vi "SimpleCalculator.vi"(1 "Operation":enum16{"ADD", "SUBTRACT", "MULTIPLY", "DIVIDE"}(ring), 2 "Number 2":dbl, 3 "Number 1":dbl) -> (0 "Result":dbl)   [LabVIEW 2020]
doc: "Simple calculator. Perform one form four mathematical operation on two numbers. Comments in polish language."
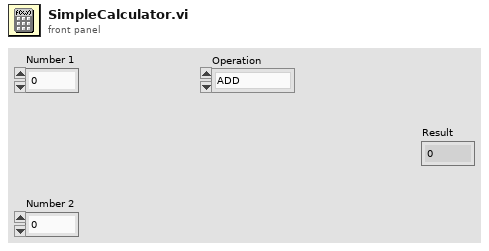
[diagram p1: front panel]
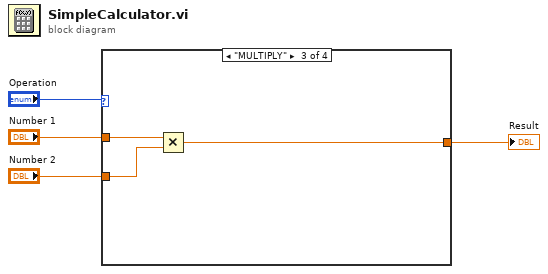
[diagram p0: block diagram]
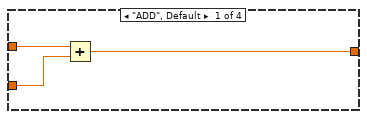
[diagram p2: hidden frame]
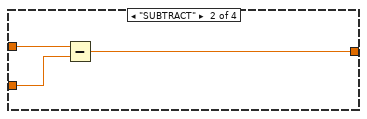
[diagram p3: hidden frame]
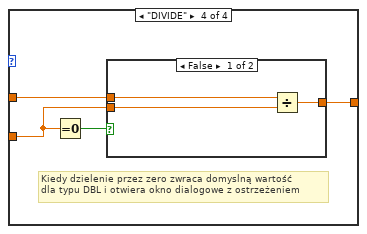
[diagram p4: hidden frame]
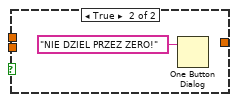
[diagram p5: hidden frame]
diagram:
  n1 = case shown="\"MULTIPLY\"" "Operation" {
    tunnel: "Number 1" -> [w7 w10 w13 w17]
    tunnel: "Number 2" -> [w6 w9 w12 w15]
    tunnel: [w5 w8 w11 w16] -> w1
    frame "ADD", Default {
      n2 = Add(x=w7, y=w6) -> (x+y=w5:dbl)
    }
    frame "SUBTRACT" {
      n3 = Subtract(x=w10, y=w9) -> (x-y=w8:dbl)
    }
    frame "MULTIPLY" {
      n4 = Multiply(x=w13, y=w12) -> (x*y=w11:dbl)
    }
    frame "DIVIDE" {
      # "Kiedy dzielenie przez zero zwraca domyslną wartość\ndla typu DBL i otwiera okno dialogowe z ostrzeżeniem"
      n5 = Equal To 0?(x=w15) -> (x = 0?=w14:bool)
      n6 = case shown="False" w14 {
        tunnel: w17 -> [w20 _]
        tunnel: [w19 _] -> w16
        tunnel: w15 -> [w18 _]
        frame False {
          n7 = Divide(x=w20, y=w18) -> (x/y=w19:dbl)
        }
        frame True {
          n8 = One Button Dialog(message="NIE DZIEL PRZEZ ZERO!") -> ()  [unwired: 1 in, 1 out]
        }
      }
    }
  }
  "Result" <- w1
